vi "DefaultTemplateMeasurement_GetUiDetails_CorrectUiPathUrl.vi"() -> (6 "pass":bool, 8 "result":string, 15 "error out":errorcluster)   [LabVIEW 2020]
uses:
  <vilib>/MeasurementLink/MeasurementLink Measurement Template/Advanced/MeasurementPlugin.lvclass
  <vilib>/MeasurementLink/MeasurementLink Measurement Template/Measurement UI.vi
  <vilib>/ErrorRing/Error Ring.xnode
  <vilib>/MeasurementLink/MeasurementLink Measurement Template/MeasurementLink Measurement Template.lvlib
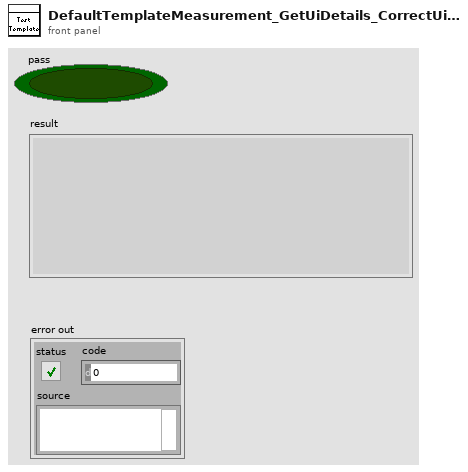
[diagram p1: front panel]
types:
  T1 = typedef "MeasurementLink Measurement Server Internal.lvlib/ni_measurementlink_measurement_v1_UserInterfaceDetails.ctl" = cluster{"file_url":string}
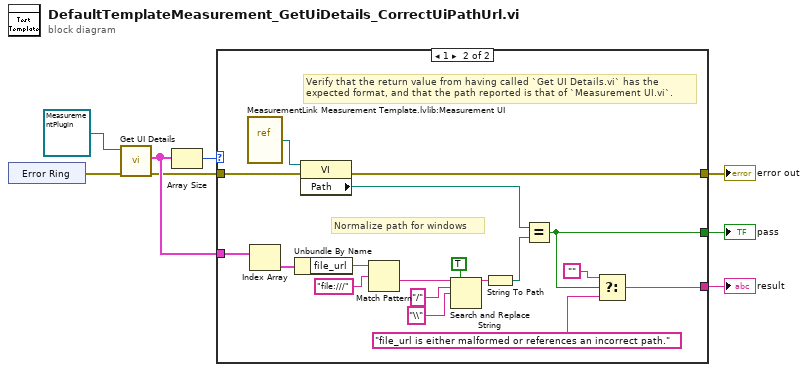
[diagram p0: block diagram]
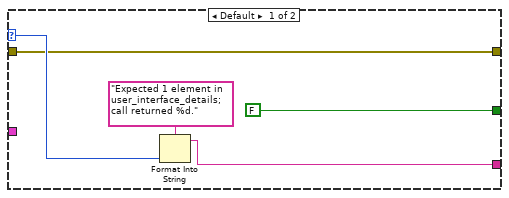
[diagram p2: hidden frame]
diagram:
  n1 = xnode "Error Ring"() -> ("error out"=w7:errorcluster)
  n2 = call-dynamic "Get UI Details.vi"("error in"=w7, "gRPC Server in"=refnum<class "MeasurementPlugin.lvclass"> refnum ("MeasurementLink Measurement Template.lvlib:MeasurementPlugin.lvclass")) -> ("error out"=w1:errorcluster, "user_interface_details"=w4:T1[])  [unwired: 7 in, 1 out]
  n3 = Array Size(array=w4) -> (size(s)=w3:i32)
  n4 = case shown="1" w3 {
    selector: w3 -> [w11 _]
    tunnel: [FALSE w19] -> w6
    tunnel: [w10 w21] -> w5
    tunnel: w4 -> [_ w31]
    tunnel: [w9 w23] -> w2
    tunnel: w1 -> [w9 w27]
    frame Default {
      n5 = Format Into String(format string="Expected 1 element in user_interface_details; call returned %d.", w11) -> (resulting string=w10:string)  [unwired: 2 in, 1 out]
    }
    frame 1 {
      # "Normalize path for windows"
      # "Verify that the return value from having called `Get UI Details.vi` has the expected format, and that the path reported is that of `Measurement UI.vi`."
      n6 = vi-ref "MeasurementLink Measurement Template.lvlib:Measurement UI.vi"() -> (w26:refnum<vi>)
      n7 = Index Array(array=w31) -> (element=w30:T1)  [unwired: 1 in]
      n8 = Unbundle By Name(w30) -> ("file_url"=w29:string)
      n9 = property class="VI"(reference=w26, error in=w27) -> (error out=w23:errorcluster, "Path"=w25:path)  [unwired: 1 out]
      n10 = Match Pattern(string=w29, regular expression="file:///" ("format string")) -> (after substring=w17:string)  [unwired: 1 in, 3 out]
      n11 = Search and Replace String(replace all?=TRUE ("replace all? (F)"), input string=w17, search string="/", replace string="\\" ("replace string (\"\")")) -> (result string=w16:string)  [unwired: 4 in, 3 out]
      n12 = String To Path(string=w16) -> (path=w24:path)
      n13 = Equal?(x=w25, y=w24) -> (x = y?=w19:bool)
      n14 = Select(t="", s=w19, f="file_url is either malformed or references an incorrect path." ("format string")) -> (s? t:f=w21:string)
    }
  }
  "error out" <- w2
  "pass" <- w6
  "result" <- w5
